vi "Apply Memory Operations.vi"(8 "error in (no error)":errorcluster, 9 "Operation (0: Data -> Memory)":i32(ring) items=["Data -> Memory", "Data + Memory", "Data - Memory", "Data * Memory", "Data / Memory"], 10 "Channel (1)":i32=1, 11 "VISA resource name":refnum<visa-resource-name>) -> (0 "error out":errorcluster, 3 "VISA resource name out":refnum<visa-resource-name>)   [LabVIEW 2018, in "Keysight PNA Series.lvlib"]
doc: "Sets math operations on the currently selected measurement and the trace stored in memory."
uses:
  Keysight PNA Series.lvlib
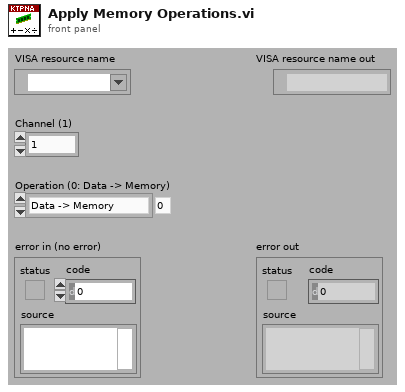
[diagram p1: front panel]
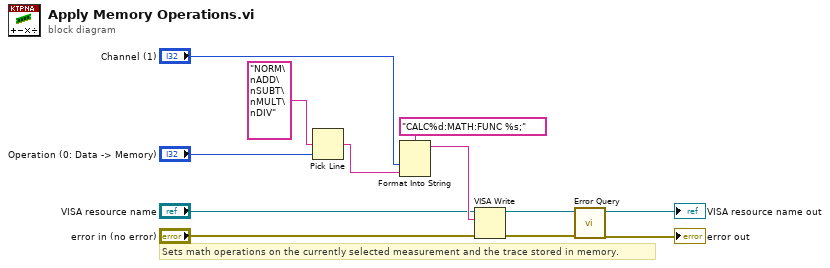
[diagram p0: block diagram]
diagram:
  # "Sets math operations on the currently selected measurement and the trace stored in memory."
  n1 = Pick Line(multi-line string="NORM\nADD\nSUBT\nMULT\nDIV", line index="Operation (0: Data -> Memory)") -> (output string=w8:string)  [unwired: 1 in]
  n2 = Format Into String(format string="CALC%d:MATH:FUNC %s;", "Channel (1)", w8) -> (resulting string=w7:string)  [unwired: 2 in, 1 out]
  n3 = VISA Write(VISA resource name="VISA resource name", write buffer=w7, error in (no error)="error in (no error)") -> (VISA resource name out=w4:refnum<visa-resource-name>, error out=w3:errorcluster)  [unwired: 1 out]
  n4 = call "Error Query.vi"("error in (no error)"=w3, "VISA resource name"=w4) -> ("error out"=→"error out":errorcluster, "VISA resource name out"=→"VISA resource name out":refnum<visa-resource-name>)  [unwired: 6 in, 2 out]
